vi "Write Config.vi"(8 "error in (no error)":errorcluster, 10 "Configuration":refnum<class "Configuration.lvclass">, 11 "LiDAR in":refnum<class "Telnet V2.lvclass">) -> (0 "error out":errorcluster, 3 "LiDAR out":refnum<class "Telnet V2.lvclass">)   [LabVIEW 2018]
uses:
  Telnet V2.lvclass
  C:/AME Test Engineering/LabVIEW/PPLs/LiDAR/Parent/LiDAR.lvlibp/LiDAR.lvclass
  PPLs/Configuration/Configuration.lvlibp/Configuration.lvclass
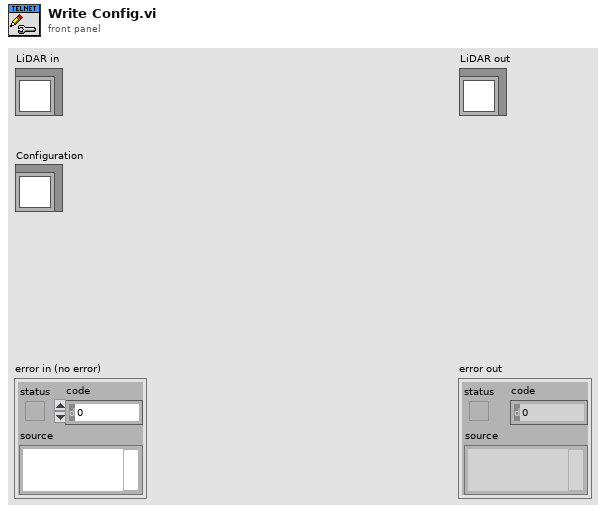
[diagram p1: front panel]
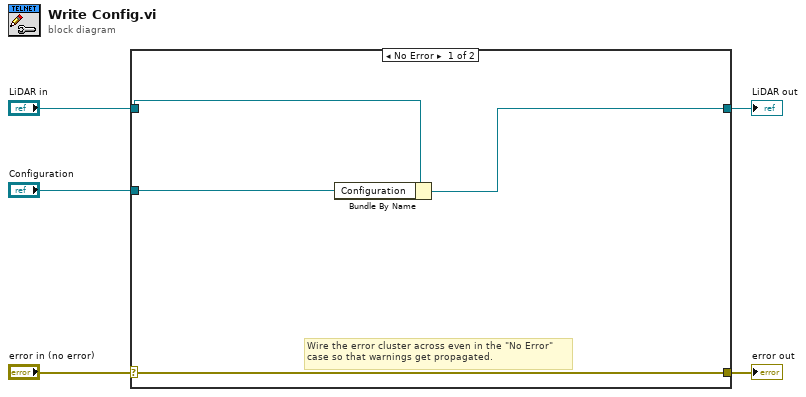
[diagram p0: block diagram]
diagram:
  n1 = case shown="No Error" "error in (no error)" {
    selector: "error in (no error)" -> [w9 w11]
    tunnel: [w9 w11] -> w4
    tunnel: [w6 w10] -> w2
    tunnel: "LiDAR in" -> [w8 w10]
    tunnel: "Configuration" -> [w7 _]
    frame No Error {
      # "Wire the error cluster across even in the \"No Error\"\ncase so that warnings get propagated."
      n2 = Bundle By Name(cluster=w8, "Configuration"=w7) -> (w6:refnum<class "Telnet V2.lvclass">)
    }
    frame Error {
    }
  }
  "error out" <- w4
  "LiDAR out" <- w2
